vi "Fade.vi"(8 "error in (no error)":errorcluster, 11 "Button in":refnum<class "Button.lvclass">) -> (0 "error out":errorcluster, 3 "Button out":refnum<class "Button.lvclass">)   [LabVIEW 2018, in "Button.lvclass"]
uses:
  Button.lvclass
  Button.lvclass/Button.ctl
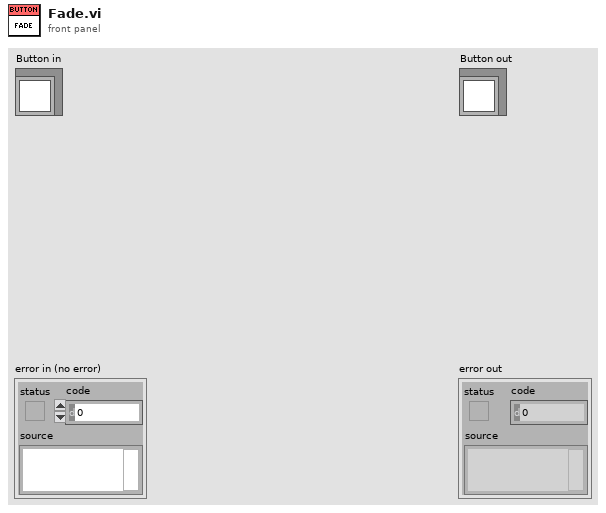
[diagram p1: front panel]
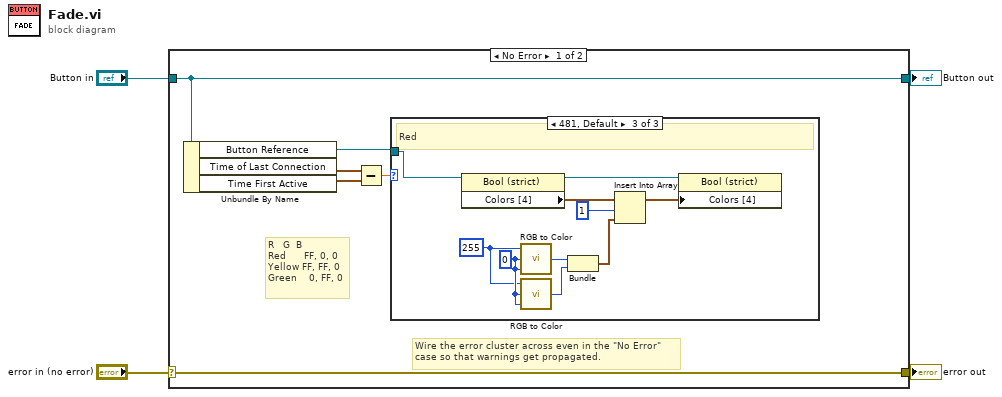
[diagram p0: block diagram]
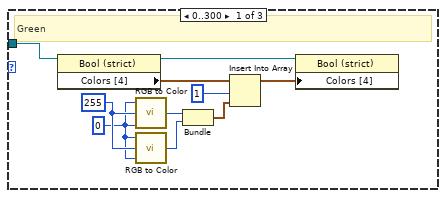
[diagram p2: hidden frame]
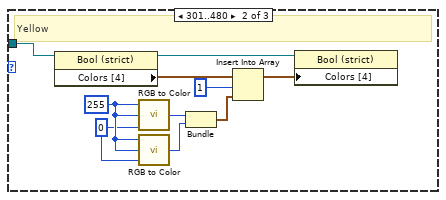
[diagram p3: hidden frame]
diagram:
  n1 = case shown="No Error" "error in (no error)" {
    selector: "error in (no error)" -> [w5 w42]
    tunnel: [w5 w42] -> w3
    tunnel: [w6 w41] -> w1
    tunnel: "Button in" -> [w6 w41]
    frame No Error {
      # "R   G  B\nRed      FF, 0, 0\nYellow FF, FF, 0\nGreen    0, FF, 0"
      # "Wire the error cluster across even in the \"No Error\"\ncase so that warnings get propagated."
      n2 = Unbundle By Name(w6) -> ("Button Reference"=w7:refnum<vi>, "Time of Last Connection"=w10:timestamp, "Time First Active"=w9:timestamp)
      n3 = Subtract(x=w10, y=w9) -> (x-y=w8:dbl)
      n4 = case shown="481, Default" w8 {
        tunnel: w7 -> [w13 w23 w32]
        frame 0..300 {
          w15 = u8 0 ("R")
          w16 = u8 255 ("R")
          # "Green"
          n5 = property class="Bool (strict)"(reference=w13) -> (reference out=w12:refnum<vi>, "Colors [4]"=w11:cluster{u32, u32}[])  [unwired: 1 in, 1 out]
          n6 = call <vilib>:"RGB to Color.vi"("B"=w15, "G"=w16, "R"=w15) -> ("Color"=w19:u32)
          n7 = call <vilib>:"RGB to Color.vi"("B"=w15, "G"=w16, "R"=w15) -> ("Color"=w18:u32)
          n8 = Bundle("Color"=w19, "Color"=w18) -> (w17:cluster{"Color":u32, "Color":u32})  [unwired: 1 in]
          n9 = Insert Into Array(array=w11, index=1, new element=w17) -> (w14:cluster{u32, u32}[])
          n10 = property class="Bool (strict)"(reference=w12, "Colors [4]"=w14) -> ()  [unwired: 1 in, 2 out]
        }
        frame 301..480 {
          w25 = u8 0 ("R")
          w26 = u8 255 ("R")
          # "Yellow"
          n11 = property class="Bool (strict)"(reference=w23) -> (reference out=w22:refnum<vi>, "Colors [4]"=w21:cluster{u32, u32}[])  [unwired: 1 in, 1 out]
          n12 = call <vilib>:"RGB to Color.vi"("B"=w25, "G"=w26, "R"=w26) -> ("Color"=w29:u32)
          n13 = call <vilib>:"RGB to Color.vi"("B"=w25, "G"=w26, "R"=w26) -> ("Color"=w28:u32)
          n14 = Bundle("Color"=w29, "Color"=w28) -> (w27:cluster{"Color":u32, "Color":u32})  [unwired: 1 in]
          n15 = Insert Into Array(array=w21, index=1, new element=w27) -> (w24:cluster{u32, u32}[])
          n16 = property class="Bool (strict)"(reference=w22, "Colors [4]"=w24) -> ()  [unwired: 1 in, 2 out]
        }
        frame 481, Default {
          w35 = u8 255 ("G")
          w36 = u8 0 ("G")
          # "Red"
          n17 = property class="Bool (strict)"(reference=w32) -> (reference out=w31:refnum<vi>, "Colors [4]"=w33:cluster{u32, u32}[])  [unwired: 1 in, 1 out]
          n18 = call <vilib>:"RGB to Color.vi"("B"=w36, "G"=w36, "R"=w35) -> ("Color"=w39:u32)
          n19 = call <vilib>:"RGB to Color.vi"("B"=w36, "G"=w36, "R"=w35) -> ("Color"=w38:u32)
          n20 = Bundle("Color"=w39, "Color"=w38) -> (w37:cluster{"Color":u32, "Color":u32})  [unwired: 1 in]
          n21 = Insert Into Array(array=w33, index=1, new element=w37) -> (w34:cluster{u32, u32}[])
          n22 = property class="Bool (strict)"(reference=w31, "Colors [4]"=w34) -> ()  [unwired: 1 in, 2 out]
        }
      }
    }
    frame Error {
    }
  }
  "error out" <- w3
  "Button out" <- w1
